vi "读取ini文件.vi"(8 "error in (no error)":errorcluster caption="错误输入（无错误）", 10 "名称":string[](array[string]), 11 "configuration file path":path caption="配置文件的路径") -> (0 "error out":errorcluster caption="错误输出", 2 "值":string[](array[string]))   [LabVIEW 2017]
doc: "读取ini文件"
uses:
  <vilib>/Utility/config.llb/Read Key (String).vi
  <vilib>/Utility/config.llb/NI_LVConfig.lvlib
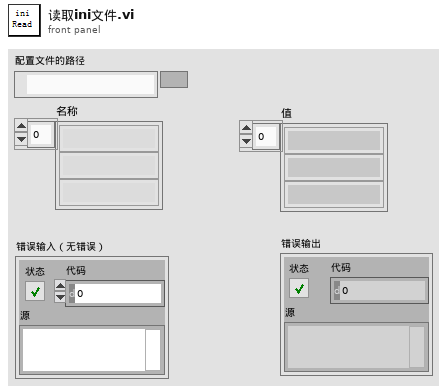
[diagram p1: front panel]
types:
  T1 = typedef "NI_LVConfig.lvlib/Config Data RefNum.ctl" = refnum<k1>
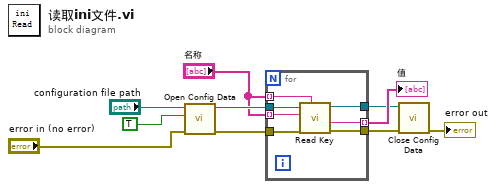
[diagram p0: block diagram]
diagram:
  n1 = call <vilib>:"Open Config Data.vi"("error in (no error)"="error in (no error)", "create file if necessary (T)"=TRUE, "configuration file path"="configuration file path") -> ("error out"=w9:errorcluster, "refnum"=w10:T1)  [unwired: 6 in, 1 out]
  n2 = for {
    tunnel: w10 -> [w17]
    tunnel: w9 -> [w16]
    tunnel: "名称" -> [w15] mode=indexing
    tunnel: "名称" -> [w14] mode=indexing
    tunnel: [w13] -> w5 mode=indexing
    tunnel: [w12] -> w4
    tunnel: [w11] -> w3
    n3 = call-poly <vilib>:"Read Key.vi"("section"=w14, "error in (no error)"=w16, "key"=w15, "refnum"=w17) -> ("error out"=w11:errorcluster, "value"=w13:string, "refnum out"=w12:T1)  [unwired: 4 in, 1 out]
  }
  "值" <- w5
  n4 = call <vilib>:"Close Config Data.vi"("error in (no error)"=w3, "refnum"=w4) -> ("error out"=→"error out":errorcluster)  [unwired: 8 in, 1 out]
